vi "Host - Thruster Drstatus Decode (SubVI).vi"(10 "Data init in":dbl[](array[numeric]), 11 "read buffer":string) -> (3 "Data init out":dbl[](array[numeric]))   [LabVIEW 2021]
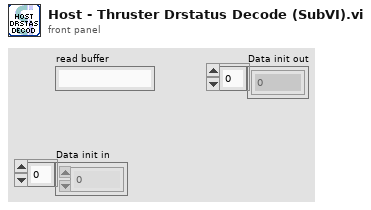
[diagram p1: front panel]
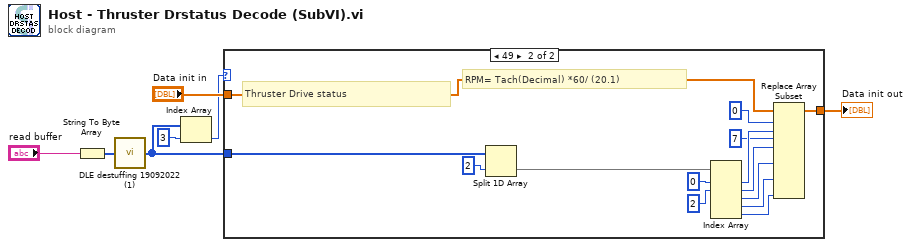
[diagram p0: block diagram]
diagram:
  n1 = String To Byte Array(string="read buffer") -> (unsigned byte array=w7:u8[])
  n2 = call "DLE destuffing 19092022 (1).vi"("DLE stuffed input"=w7) -> ("DLE destuffed output"=w6:u8[])  [unwired: 4 in]
  n3 = Index Array(array=w6, index=3) -> (element=w3:u8)
  n4 = case shown="49" w3 {
    tunnel: w6 -> [_ w19]
    tunnel: [w8 w15] -> w5
    tunnel: "Data init in" -> [w8 w18]
    frame 0, Default {
    }
    frame 49 {
      # "RPM= Tach(Decimal) *60/ (20.1)"
      # "Thruster Drive status"
      n5 = Split 1D Array(array=w19, index=2) -> (second subarray=w22:u8[])  [unwired: 1 out]
      n6 = Index Array(array=w22, index #1=0 ("index"), index #2=2 ("index")) -> (element #1=w16:u8, element #2=w12:u8, element #3=w9:u8, element #4=w11:u8, element #5=w10:u8)  [unwired: 3 in]
      n7 = Replace Array Subset(array=w18, new element #1=w16, index #1=0 ("index"), new element #2=w12, index #2=7 ("index"), new element #3=w9, new element #4=w11, new element #5=w10) -> (w15:dbl[])  [unwired: 3 in]
    }
  }
  "Data init out" <- w5
